vi "AppendTableToReport_SFP_86To85.vi"(9 "Scratchpad Diagram (Contains XNode)":refnum<vi>, 10 "XRef (Scratchpad Diagram)":refnum<vi>, 11 "XRef (Original Diagram)":refnum<vi>) -> (1 "Custom Label":string, 2 "Custom Warning To Issue":string, 3 "Action":T1)   [LabVIEW 2020]
uses:
  <vilib>/XSFPSupport/SFPReplaceAction.ctl
  <vilib>/XSFPSupport/NI_XSFPSupport.lvlib
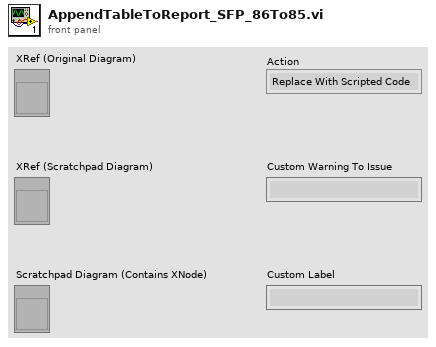
[diagram p1: front panel]
types:
  T1 = typedef "NI_XSFPSupport.lvlib/SFPReplaceAction.ctl" = enum32{"Replace With Scripted Code", "Replace With Label", "Fail SFP"}
  T2 = typedef "LVPositionTypeDef.ctl" = cluster{"Left":i32, "Top":i32}
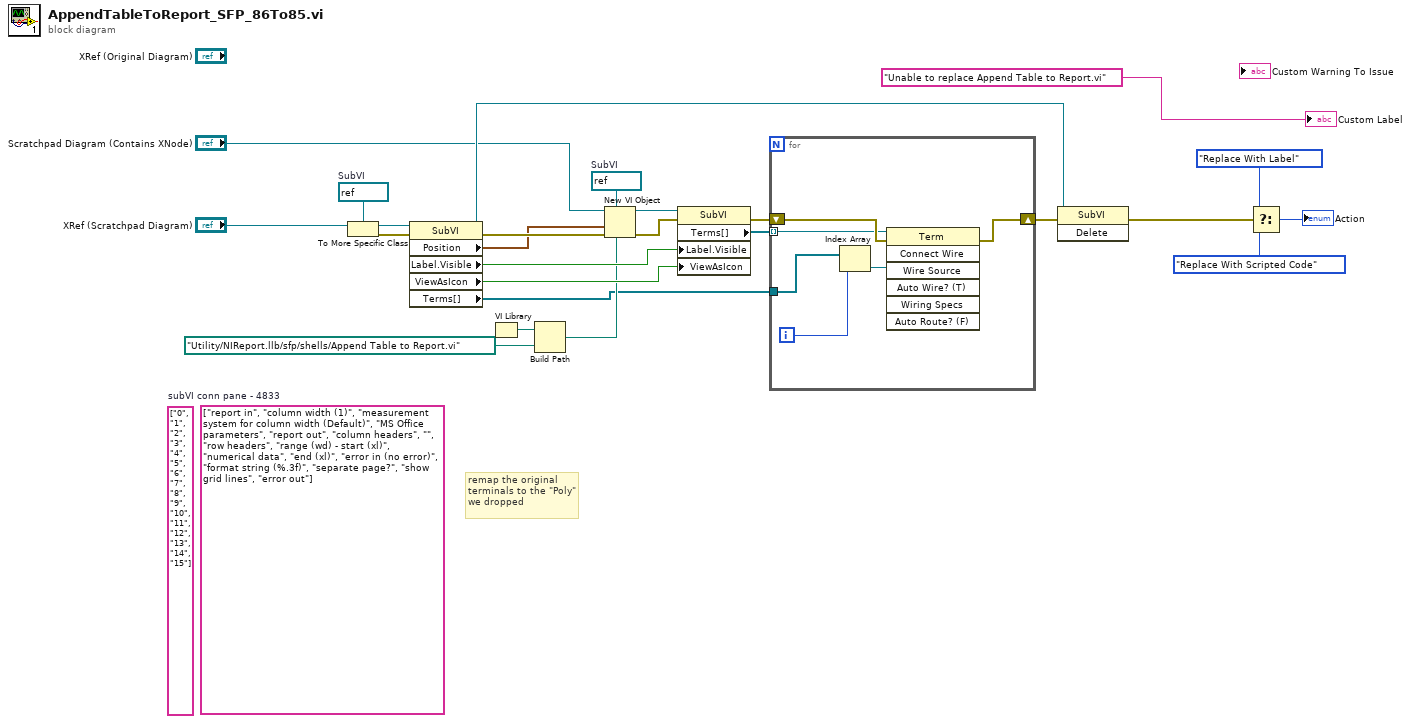
[diagram p0: block diagram]
diagram:
  (unwired) string[] ["0", "1", "2", "3", "4", "5", "6", "7", "8", "9", "10", "11", "12", "13", "14", "15"]
  (unwired) string[] ["report in", "column width (1)", "measurement system for column width (Default)", "MS Office parameters", "report out", "column headers", "", "row headers", "range (wd) - start (xl)", "numerical data", "end (xl)", "error in (no error)", "format string (%.3f)", "separate page?", "show grid lines", "error out"]  # subVI conn pane - 4833
  w15 = refnum<vi> refnum  # SubVI
  w18 = refnum<vi> refnum  # SubVI
  # "remap the original terminals to the \"Poly\" we dropped"
  n1 = To More Specific Class(target class=w18, reference="XRef (Scratchpad Diagram)") -> (specific class reference=w17:refnum<vi>, error out=w25:errorcluster)  [unwired: 1 in]
  n2 = property class="SubVI"(reference=w17, error in=w25) -> (reference out=w5:refnum<vi>, error out=w24:errorcluster, "Position"=w16:T2, "Label.Visible"=w13:bool, "ViewAsIcon"=w12:bool, "Terms[]"=w2:refnum<vi>[])
  n3 = VI Library() -> (path=w7:path)
  n4 = Build Path(base path=w7, name or relative path=path "Utility/NIReport.llb/sfp/shells/Append Table to Report.vi") -> (appended path=w4:path)
  n5 = New VI Object(vi object class=w15, owner refnum="Scratchpad Diagram (Contains XNode)", position/next to=w16, 6:w4, 8:w24) -> (object refnum=w14:refnum<vi>, 0:w23:errorcluster)  [unwired: 3 out]
  n6 = property class="SubVI"(reference=w14, error in=w23, "Label.Visible"=w13, "ViewAsIcon"=w12) -> (error out=w22:errorcluster, "Terms[]"=w1:refnum<vi>[])  [unwired: 1 out]
  n7 = for {
    tunnel: w1 -> [w29] mode=indexing
    tunnel: w2 -> [w27]
    shift-right: [w30] -> w21
    shift-left: w22 -> [w31]
    i -> [w28]
    n8 = Index Array(array=w27, index=w28) -> (element=w26:refnum<vi>)
    n9 = invoke class="Term" method="Connect Wire"(reference=w29, error in=w31, "Wire Source"=w26) -> (error out=w30:errorcluster)  [unwired: 4 in, 6 out]
  }
  n10 = invoke class="SubVI" method="Delete"(reference=w5, error in=w21) -> (error out=w20:errorcluster)  [unwired: 1 in, 2 out]
  n11 = Select(t=SFPReplaceAction."Replace With Label" ("Action"), s=w20, f=SFPReplaceAction."Replace With Scripted Code" ("Action")) -> (s? t:f=→"Action":T1)
  "Custom Label" <- "Unable to replace Append Table to Report.vi" ("Custom Label")
